vi "getAllChannels.vi"(8 "error in (no error)":errorcluster, 11 "device in":refnum<class "device.lvclass">) -> (0 "error out":errorcluster, 2 "ChannelArray":refnum<class "ChannelArray.lvclass">, 3 "device out":refnum<class "device.lvclass">)   [LabVIEW 2009, in "Tools.lvlib" / "DatabaseHelpers.lvlib" / "device.lvclass"]
uses:
  device.lvclass
  ChannelArray/ChannelArray.lvclass
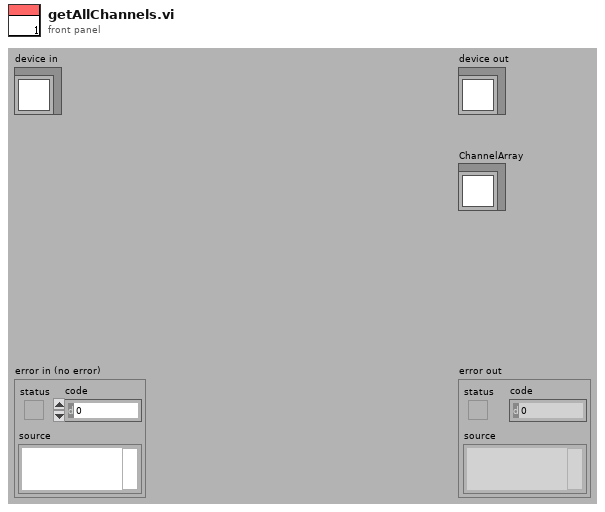
[diagram p1: front panel]
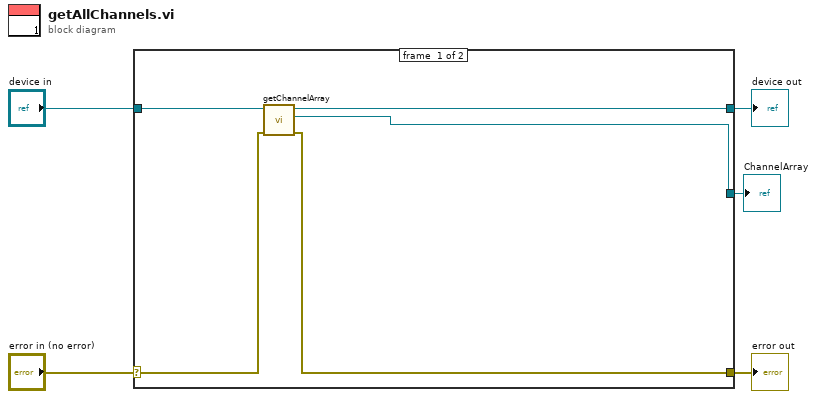
[diagram p0: block diagram]
diagram:
  n1 = case shown="No Error" "error in (no error)" {
    selector: "error in (no error)" -> [w7 w12]
    tunnel: [w6 w12] -> w4
    tunnel: [w9 w11] -> w2
    tunnel: "device in" -> [w10 w11]
    tunnel: [w8 _] -> w1
    frame #0 {
      n2 = call "getChannelArray.vi"("error in (no error)"=w7, "device.lvclass in"=w10) -> ("error out"=w6:errorcluster, "ChannelArray.lvclass"=w8:refnum<class "ChannelArray.lvclass">, "device.lvclass out"=w9:refnum<class "device.lvclass">)  [unwired: 7 in]
    }
    frame #1 {
    }
  }
  "error out" <- w4
  "device out" <- w2
  "ChannelArray" <- w1
